vi "SaveErrorLog.vi"(8 "Error In":errorcluster) -> (0 "error out":errorcluster)   [LabVIEW 2019]
uses:
  <vilib>/Utility/file.llb/Write Delimited Spreadsheet (string).vi
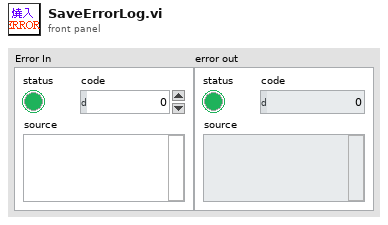
[diagram p1: front panel]
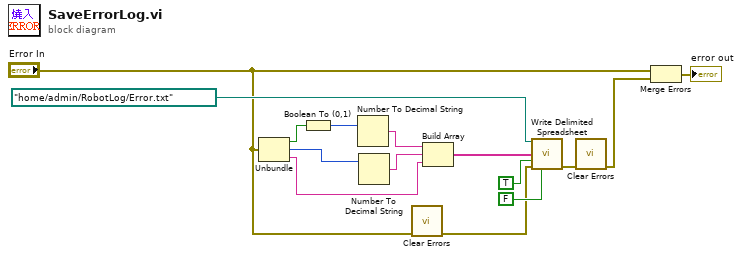
[diagram p0: block diagram]
diagram:
  n1 = Unbundle("Error In") -> ("status"=w15:bool, "code"=w13:i32, "source"=w10:string)
  n2 = Boolean To (0,1)(Boolean=w15) -> (0, 1=w14:i16)
  n3 = Number To Decimal String(number=w14) -> (decimal integer string=w12:string)  [unwired: 1 in]
  n4 = Number To Decimal String(number=w13) -> (decimal integer string=w11:string)  [unwired: 1 in]
  n5 = call <vilib>:"Clear Errors.vi"("error in (no error)"="Error In") -> ("error out"=w1:errorcluster)  [unwired: 5 in, 1 out]
  n6 = Build Array(w12, w11, w10) -> (w9:string[])
  n7 = call-poly <vilib>:"Write Delimited Spreadsheet.vi"("file path (dialog if empty)"=path "/home/admin/RobotLog/Error.txt", "1D data"=w9, "append to file? (new file:F)"=TRUE, "error in (no error)"=w1, "transpose? (no:F)"=FALSE) -> ("error out"=w8:errorcluster)  [unwired: 9 in, 1 out]
  n8 = call <vilib>:"Clear Errors.vi"("error in (no error)"=w8) -> ("error out"=w7:errorcluster)  [unwired: 5 in, 1 out]
  n9 = Merge Errors("Error In", w7) -> (→"error out":errorcluster)
